vi "Icc_Vca.vi"(0 "VetorDeDados":dbl[][](array[numeric]), 1 "pontos":dbl) -> (6 "Icc":dbl, 7 "Vca":dbl, 8 "Pmp":dbl)   [LabVIEW 2012]
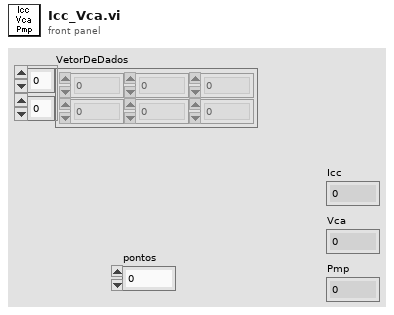
[diagram p1: front panel]
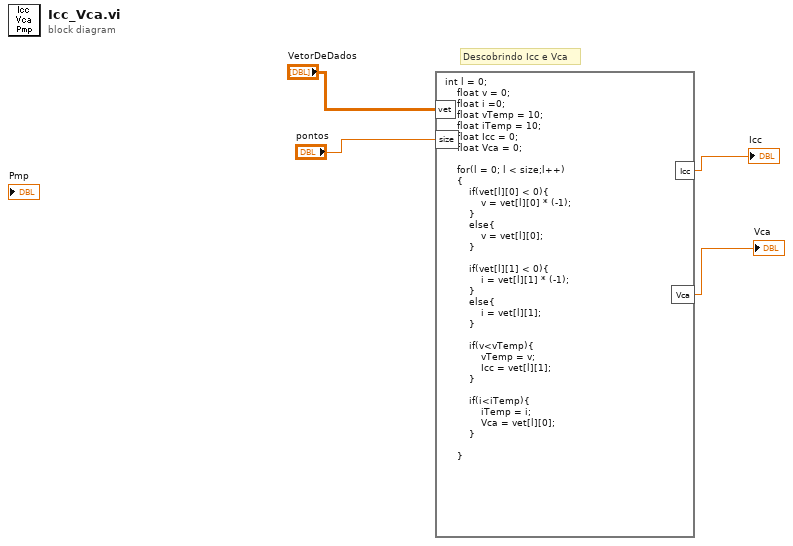
[diagram p0: block diagram]
diagram:
  # "Descobrindo Icc e Vca"
  n1 = formula code="int l = 0;\n    float v = 0;\n    float i =0;\n    float vTemp = 10;\n    float iTemp = 10;\n    float Icc = 0;\n    float Vca = 0;\n\n    for(l = 0; l < size;l++)\n    {\n        if(vet[l][0] < 0){\n            v = vet[l][0] * (-1);\n        }\n        else{\n            v = vet[l][0];\n        }\n\n        if(vet[l][1] < 0){\n            i = vet[l][1] * (-1);\n        }\n        else{\n            i = vet[l][1];\n        }\n\n        if(v<vTemp){\n            vTemp = v;\n            Icc = vet[l][1];\n        }\n\n        if(i<iTemp){\n            iTemp = i;\n            Vca = vet[l][0];\n        }\n\n    }"("vet"="VetorDeDados", "size"="pontos") -> ("Icc"=→"Icc":dbl, "Vca"=→"Vca":dbl)
